vi "NT Globals.vi"() -> ()   [LabVIEW 2017]
panel:
  in  "Write Operations":i32
  in  "Read Operations":i32
  in  "Bytes Transmitted":i32
  in  "Updates":i32
  in  "Start Time":timestamp
  in  "Variable Count":i32
  in  "Name":string
  in  "Produce Read Errors":bool
  in  "Server Connection":refnum<k5>
  in  "IsClient":bool
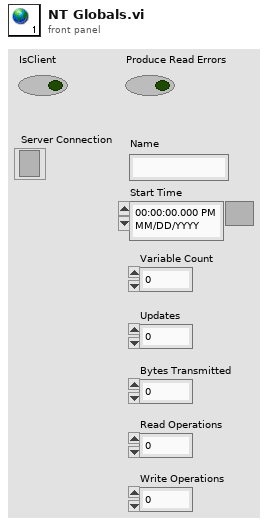
[diagram p1: front panel]
diagram:
